vi "Get GObject by ID.vi"(8 "error in (no error)":errorcluster, 10 "ID":i32, 11 "Data Cluster in":T1) -> (0 "error out":errorcluster, 2 "gobject":refnum<vi>, 3 "Data Cluster out":T1)   [LabVIEW 2025, in "Scripting Server.lvlib"]
uses:
  Scripting Server.lvlib
  Module Data--cluster.ctl
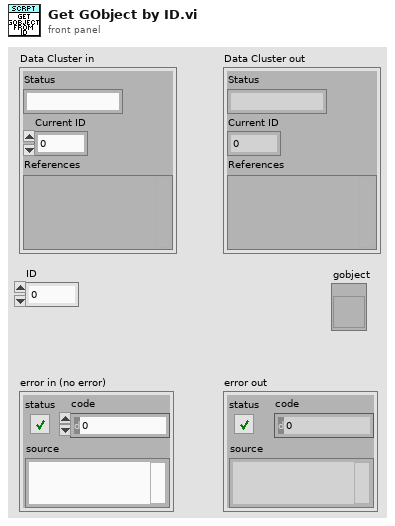
[diagram p1: front panel]
types:
  T1 = typedef "Scripting Server.lvlib/Module Data--cluster.ctl" = cluster{"Status":string, "Current ID":i32, "References":variant}
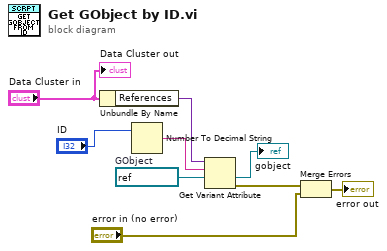
[diagram p0: block diagram]
diagram:
  w4 = refnum<vi> refnum  # GObject
  n1 = Unbundle By Name("Data Cluster in") -> ("References"=w7:variant)
  n2 = Number To Decimal String(number="ID") -> (decimal integer string=w8:string)  [unwired: 1 in]
  n3 = Get Variant Attribute(Variant=w7, name=w8, default value (empty Variant)=w4) -> (value=→"gobject":refnum<vi>, error out=w9:errorcluster)  [unwired: 1 in, 2 out]
  n4 = Merge Errors(w9, "error in (no error)") -> (→"error out":errorcluster)
  "Data Cluster out" <- "Data Cluster in"
